vi "Edgertronic-get_current_settings.vi"(3 "error in (no error)":errorcluster, 5 "URL":string="192.168.1.101") -> (0 "error out":errorcluster, 1 "Current Settings:":T1={"Connection Information:"="", "Requested Genlock "="20140911165611", "Min Frame Clocks "="20140911165611", "Is Seq Clk Freq "="20140911165611", "Pretrigger Frames "="20140911165611", "Duration "="20140911165611", "Overclock "="20140911165611", "Requested Horizontal "="20140911165611", "Frames "="20140911165611", "Requested Pretrigger "="20140911165611", "Words per Frame "="20140911165611", "Buffer End "="20140911165611", "Clocks per Frame  "="20140911165611", "Requested Duration "="20140911165611", "Pretrigger "="20140911165611", "Post-trigger Frames "="20140911165611", "Vertical "="20140911165611", "Requested Vertical "="20140911165611", "Reqested Frame Rate "="20140911165611", "Frame Rate "="20140911165611", "Horizontal "="20140911165611", "Clocks per Exposure "="20140911165611", "Digital Gain "="20140911165611", "Exposure "="20140911165611", "Genlock "="20140911165611", "Analog Gain "="20140911165611", "Subsample "="20140911165611", "Requested Exposure "="20140911165611", "Iso "="20140911165611", "Requested Overclock "="20140911165611", "Requested Subsample "="20140911165611", "Requested Iso"="20140911165611", "FPGA Temp"="20140911165611", "Posttrigger Duration"="20140911165611", "dacvrefadc"="20140911165611", "Is Temp"="20140911165611", "Pretrigger Duration"="20140911165611"})   [LabVIEW 2015]
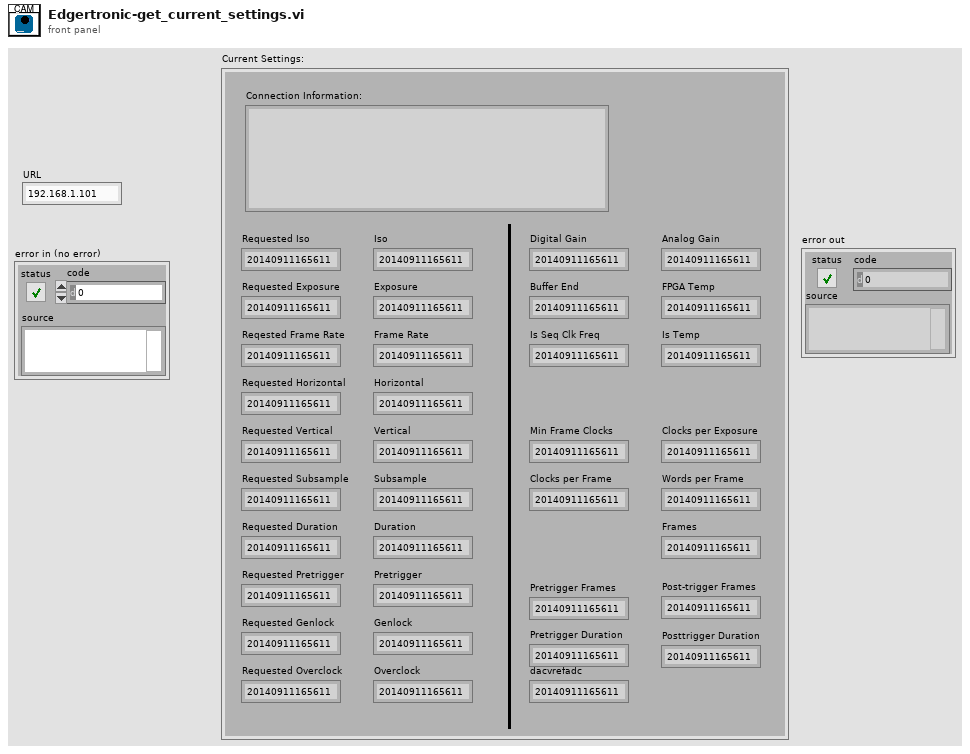
[diagram p1: front panel]
types:
  T1 = cluster{"Connection Information:":string, "Requested Genlock ":string, "Min Frame Clocks ":string, "Is Seq Clk Freq ":string, "Pretrigger Frames ":string, "Duration ":string, "Overclock ":string, "Requested Horizontal ":string, "Frames ":string, "Requested Pretrigger ":string, "Words per Frame ":string, "Buffer End ":string, "Clocks per Frame  ":string, "Requested Duration ":string, "Pretrigger ":string, "Post-trigger Frames ":string, "Vertical ":string, "Requested Vertical ":string, "Reqested Frame Rate ":string, "Frame Rate ":string, "Horizontal ":string, "Clocks per Exposure ":string, "Digital Gain ":string, "Exposure ":string, "Genlock ":string, "Analog Gain ":string, "Subsample ":string, "Requested Exposure ":string, "Iso ":string, "Requested Overclock ":string, "Requested Subsample ":string, "Requested Iso":string, "FPGA Temp":string, "Posttrigger Duration":string, "dacvrefadc":string, "Is Temp":string, "Pretrigger Duration":string}
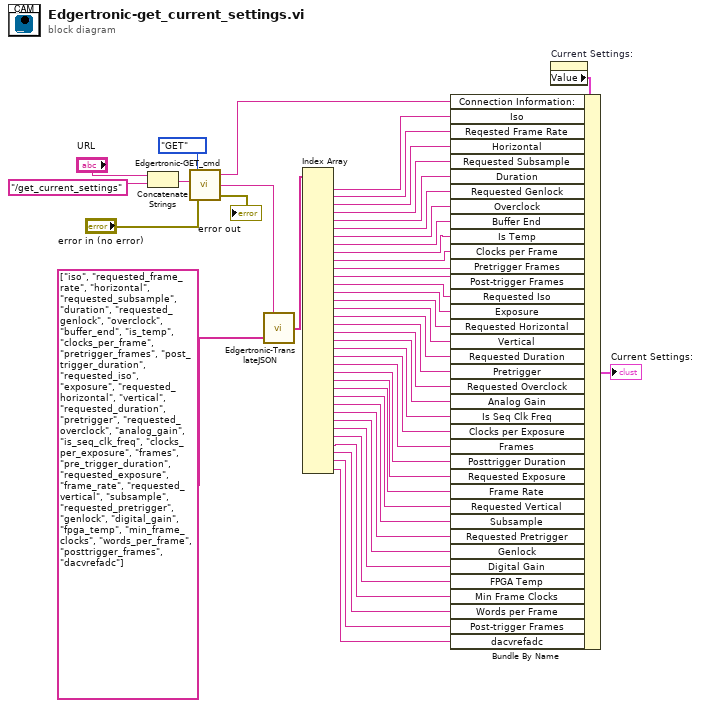
[diagram p0: block diagram]
diagram:
  n1 = Concatenate Strings("URL", "/get_current_settings" ("GET Command")) -> (w3:string)
  n2 = call "Edgertronic-GET_cmd.vi"("error in (no error)"="error in (no error)", "URL"=w3, "Type"=enum16{"GET", "POST"}."GET") -> ("error out"=→"error out":errorcluster, "data"=w42:string, "Connection Info"=w43:string)  [unwired: 1 in]
  n3 = call "Edgertronic-TranslateJSON.vi"("Commands"=string[] ["iso", "requested_frame_rate", "horizontal", "requested_subsample", "duration", "requested_genlock", "overclock", "buffer_end", "is_temp", "clocks_per_frame", "pretrigger_frames", "post_trigger_duration", "requested_iso", "exposure", "requested_horizontal", "vertical", "requested_duration", "pretrigger", "requested_overclock", "analog_gain", "is_seq_clk_freq", "clocks_per_exposure", "frames", "pre_trigger_duration", "requested_exposure", "frame_rate", "requested_vertical", "subsample", "requested_pretrigger", "genlock", "digital_gain", "fpga_temp", "min_frame_clocks", "words_per_frame", "posttrigger_frames", "dacvrefadc"] ("Array"), "data"=w42) -> ("Values"=w47:string[])  [unwired: 3 in]
  n4 = Index Array(array=w47) -> (element #1=w46:string, element #2=w40:string, element #3=w39:string, element #4=w38:string, element #5=w37:string, element #6=w36:string, element #7=w35:string, element #8=w34:string, element #9=w33:string, element #10=w32:string, element #11=w31:string, element #12=w30:string, element #13=w29:string, element #14=w28:string, element #15=w27:string, element #16=w26:string, element #17=w25:string, element #18=w24:string, element #19=w23:string, element #20=w22:string, element #21=w21:string, element #22=w20:string, element #23=w19:string, element #24=w18:string, element #25=w17:string, element #26=w16:string, element #27=w15:string, element #28=w14:string, element #29=w13:string, element #30=w12:string, element #31=w11:string, element #32=w10:string, element #33=w9:string, element #34=w8:string, element #35=w7:string, element #36=w6:string)  [unwired: 36 in]
  n5 = property on="Current Settings:" class="Clust (strict)"() -> ("Value"=w45:T1)  [unwired: 2 in, 2 out]
  n6 = Bundle By Name(cluster=w45, "Connection Information:"=w43, "Iso"=w46, "Reqested Frame Rate"=w40, "Horizontal"=w39, "Requested Subsample"=w38, "Duration"=w37, "Requested Genlock"=w36, "Overclock"=w35, "Buffer End"=w34, "Is Temp"=w33, "Clocks per Frame"=w32, "Pretrigger Frames"=w31, "Post-trigger Frames"=w30, "Requested Iso"=w29, "Exposure"=w28, "Requested Horizontal"=w27, "Vertical"=w26, "Requested Duration"=w25, "Pretrigger"=w24, "Requested Overclock"=w23, "Analog Gain"=w22, "Is Seq Clk Freq"=w21, "Clocks per Exposure"=w20, "Frames"=w19, "Posttrigger Duration"=w18, "Requested Exposure"=w17, "Frame Rate"=w16, "Requested Vertical"=w15, "Subsample"=w14, "Requested Pretrigger"=w13, "Genlock"=w12, "Digital Gain"=w11, "FPGA Temp"=w10, "Min Frame Clocks"=w9, "Words per Frame"=w8, "Post-trigger Frames"=w7, "dacvrefadc"=w6) -> (→"Current Settings:":T1)
